vi "Set Show Sent Messages.vi"(8 "error in (no error)":errorcluster, 10 "Show Sent Messages?":bool, 11 "Chronological List In":refnum<class "Chronological List.lvclass">) -> (0 "error out":errorcluster, 3 "Chronological List Out":refnum<class "Chronological List.lvclass">)   [LabVIEW 2020, in "Chronological List.lvclass"]
uses:
  Chronological List.lvclass
  Chronological List.lvclass/Chronological List.ctl
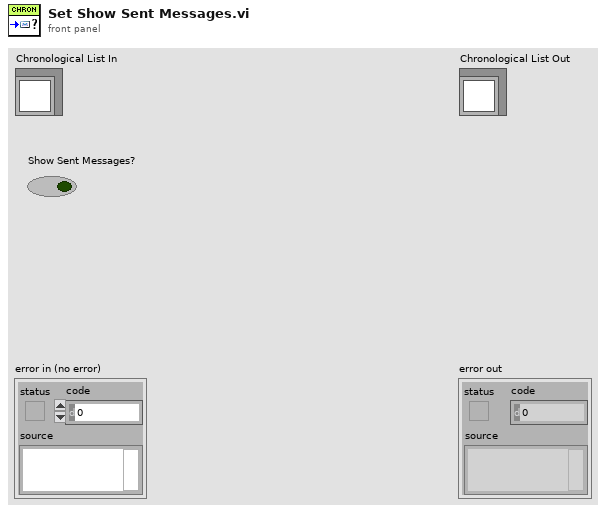
[diagram p1: front panel]
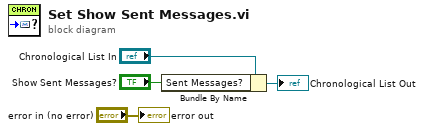
[diagram p0: block diagram]
diagram:
  n1 = Bundle By Name(cluster="Chronological List In", "Sent Messages?"="Show Sent Messages?") -> (→"Chronological List Out":refnum<class "Chronological List.lvclass">)
  "error out" <- "error in (no error)"
